vi "4.7.1.vi"() -> ()   [LabVIEW 2017]
panel:
  in  "stop":bool
  out "Waveform Chart":dbl(graph)
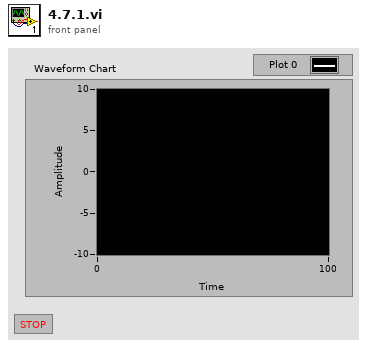
[diagram p1: front panel]
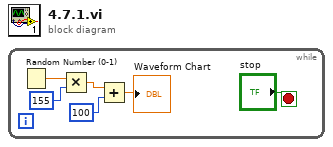
[diagram p0: block diagram]
diagram:
  n1 = while {
    stop <- "stop" stop-if-true
    n2 = Random Number (0-1)() -> (number: 0 to 1=w5:dbl)
    n3 = Multiply(x=w5, y=155) -> (x*y=w3:dbl)
    n4 = Add(x=w3, y=100) -> (x+y=→"Waveform Chart":dbl)
  }
